vi "Information.vi"(8 "error in (no error)":errorcluster, 9 "Context":T1, 10 "Information":refnum<class "Information.lvclass">, 11 "Log Record in":refnum<class "Log Record.lvclass">) -> (0 "error out":errorcluster, 3 "Log Record out":refnum<class "Log Record.lvclass">)   [LabVIEW 2021, in "Log Record.lvclass"]
uses:
  Log Record.lvclass
  Publish-Subscribe/Interfaces/Information/Information.lvclass
  Publish-Subscribe/Context.ctl
  NHMFL_Core/Libraries/Instruments/Results/Acquired Result/Acquired Result.lvclass
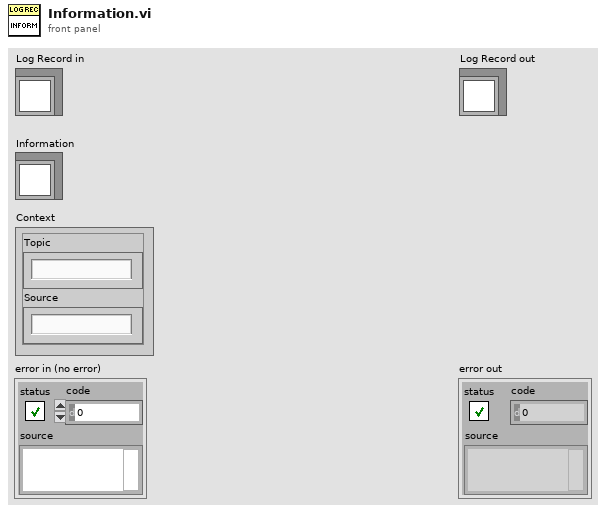
[diagram p1: front panel]
types:
  T1 = typedef "Context.ctl" = cluster{"Topic":string, "Source":string}
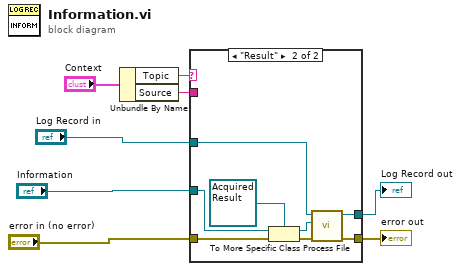
[diagram p0: block diagram]
diagram:
  n1 = Unbundle By Name("Context") -> ("Topic"=w7:string, "Source"=w8:string)
  n2 = case shown="\"Result\"" w7 {
    tunnel: "Information" -> [_ w17]
    tunnel: "error in (no error)" -> [w9 w16]
    tunnel: "Log Record in" -> [w10 w13]
    tunnel: [w10 w14] -> w1
    tunnel: [w9 w11] -> w2
    tunnel: w8 -> [_ _]
    frame "", Default {
    }
    frame "Result" {
      n3 = To More Specific Class(target class=refnum<class "Acquired Result.lvclass"> refnum ("Acquired Result.lvclass"), reference=w17, error in=w16) -> (specific class reference=w15:refnum<class "Acquired Result.lvclass">, error out=w12:errorcluster)
      n4 = call-dynamic "Process File.vi"("error in (no error)"=w12, "Result in"=w15, "Log Record in"=w13) -> ("error out"=w11:errorcluster, "Log Record out"=w14:refnum<class "Log Record.lvclass">)  [unwired: 6 in, 1 out]
    }
  }
  "error out" <- w2
  "Log Record out" <- w1
